vi "WPI_ADI_IMU_KalmanPitchRollYaw.vi"(6 "Reset?":bool, 7 "dt (ms)":dbl, 8 "Beta":dbl, 9 "Data":dbl[](array[numeric])) -> (3 "Output":dbl[](array[numeric]))   [LabVIEW 2015]
panel:
  out "output array":dbl[](array[numeric])
  out "Roll":dbl
  out "Pitch":dbl
  out "Yaw":dbl
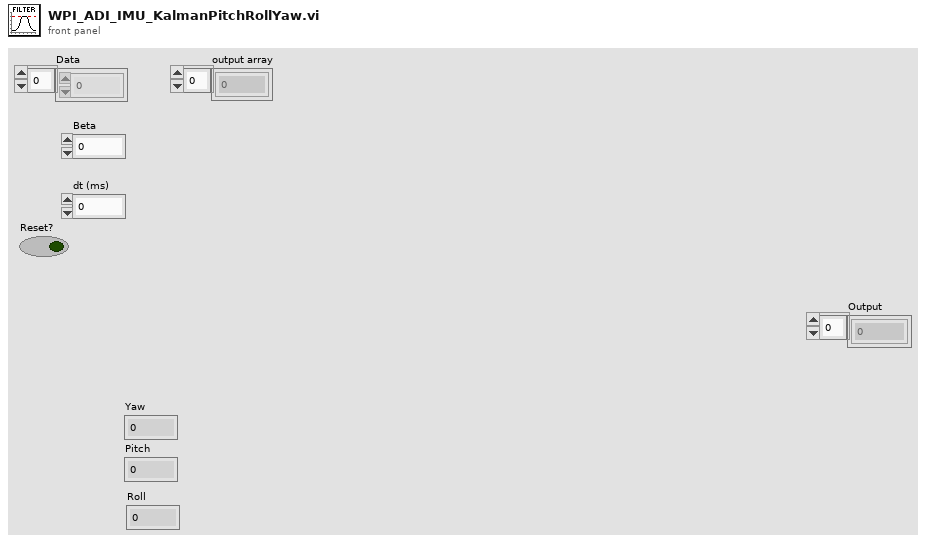
[diagram p1: front panel]
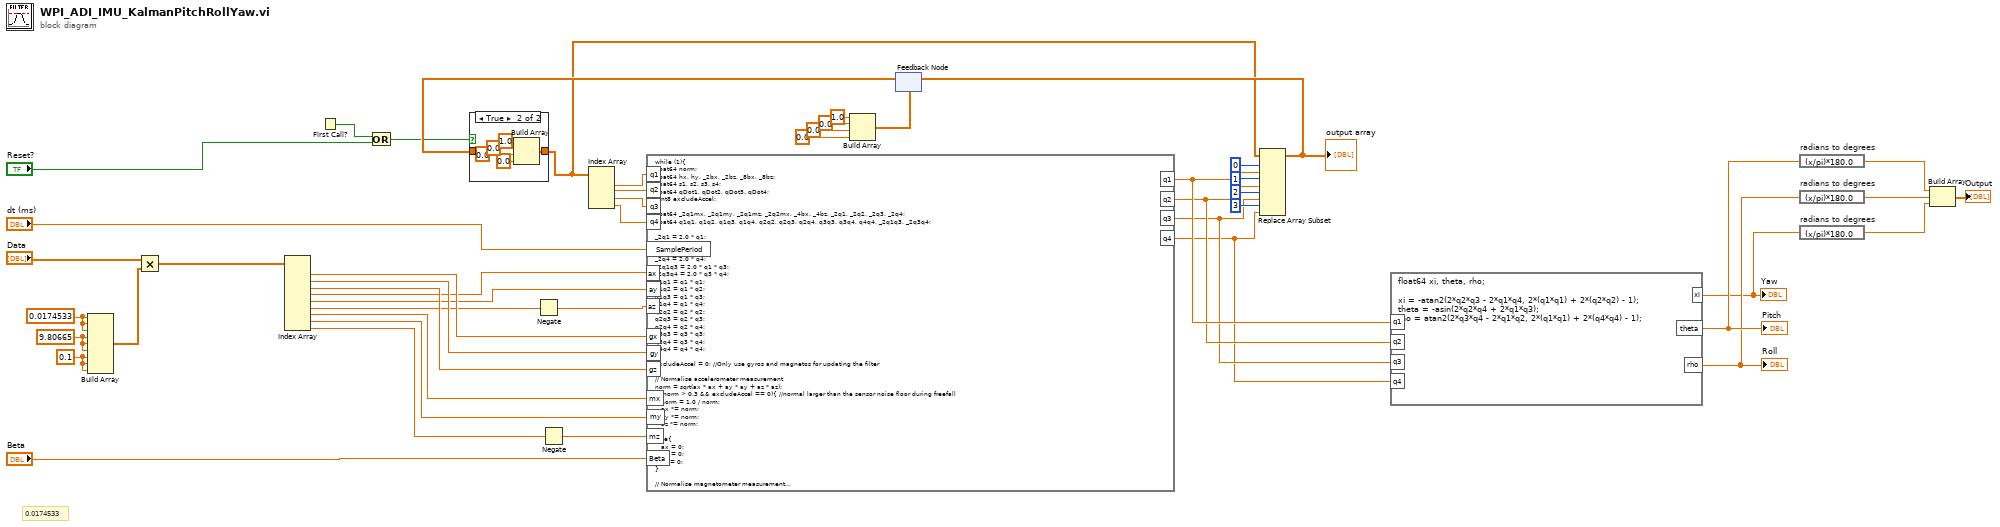
[diagram p0: block diagram]
diagram:
  w33 = 0.1
  w34 = 9.80665
  w35 = 0.0174533
  # "0.0174533"
  n1 = Build Array(w35, w35, w35, w34, w34, w34, w33, w33, w33) -> (w36:dbl[])
  n2 = Multiply(x="Data", y=w36) -> (x*y=w32:dbl[])
  n3 = Index Array(array=w32) -> (element #1=w49:dbl, element #2=w48:dbl, element #3=w47:dbl, element #4=w46:dbl, element #5=w45:dbl, element #6=w5:dbl, element #7=w1:dbl, element #8=w2:dbl, element #9=w4:dbl)  [unwired: 9 in]
  n4 = First Call?() -> (First Call?: T/F=w15:bool)
  n5 = Or(x=w15, y="Reset?") -> (x .or. y?=w16:bool)
  n6 = Negate(x=w5) -> (-x=w6:dbl)
  n7 = Negate(x=w4) -> (-x=w3:dbl)
  n8 = Build Array(1.0 ("element"), 0.0 ("element"), 0.0 ("element"), 0.0 ("element")) -> (w38:dbl[])
  n9 = feedback #1(w38) -> (w18:dbl[])
  n10 = case shown="True" w16 {
    tunnel: w18 -> [w50 _]
    tunnel: [w50 w51] -> w17
    frame False {
    }
    frame True {
      n11 = Build Array(1.0 ("element"), 0.0 ("element"), 0.0 ("element"), 0.0 ("element")) -> (w51:dbl[])
    }
  }
  n12 = Index Array(array=w17) -> (element #1=w31:dbl, element #2=w30:dbl, element #3=w29:dbl, element #4=w28:dbl)  [unwired: 4 in]
  n13 = formula code="while (1){\nfloat64 norm;\nfloat64 hx, hy, _2bx, _2bz, _8bx, _8bz;\nfloat64 s1, s2, s3, s4;\nfloat64 qDot1, qDot2, qDot3, qDot4;\nuInt8 excludeAccel;\n\nfloat64 _2q1mx, _2q1my, _2q1mz, _2q2mx, _4bx, _4bz, _2q1, _2q2, _2q3, _2q4;\nfloat64 q1q1, q1q2, q1q3, q1q4, q2q2, q2q3, q2q4, q3q3, q3q4, q4q4, _2q1q3, _2q3q4;\n\n_2q1 = 2.0 * q1;\n_2q2 = 2.0 * q2;\n_2q3 = 2.0 * q3;\n_2q4 = 2.0 * q4;\n_2q1q3 = 2.0 * q1 * q3;\n_2q3q4 = 2.0 * q3 * q4;\nq1q1 = q1 * q1;\nq1q2 = q1 * q2;\nq1q3 = q1 * q3;\nq1q4 = q1 * q4;\nq2q2 = q2 * q2;\nq2q3 = q2 * q3;\nq2q4 = q2 * q4;\nq3q3 = q3 * q3;\nq3q4 = q3 * q4;\nq4q4 = q4 * q4;\n\nexcludeAccel = 0; //Only use gyros and magnetos for updating the filter\n\n// Normalise accelerometer measurement\nnorm = sqrt(ax * ax + ay * ay + az * az);\nif (norm > 0.3 && excludeAccel == 0){ //normal larger than the sensor noise floor during freefall\n   norm = 1.0 / norm; \n   ax *= norm;\n   ay *= norm;\n   az *= norm;\n}\nelse{\n   ax = 0;\n   ay = 0;\n   az = 0;\n}\n\n// Normalise magnetometer measurement\nnorm = sqrt(mx * mx + my * my + mz * mz);\nif (norm > 0.0){\n   norm = 1.0 / norm;\n   mx *= norm;\n   my *= norm;\n   mz *= norm;\n}\nelse{\n  break; //something is wrong with the magneto readouts\n}\n\n// Reference direction of Earth's magnetic field\n_2q1mx = 2 * q1 * mx;\n_2q1my = 2 * q1 * my;\n_2q1mz = 2 * q1 * mz;\n_2q2mx = 2 * q2 * mx;\n\nhx = mx * q1q1 - _2q1my * q4 + _2q1mz * q3 + mx * q2q2 + _2q2 * my * q3 + _2q2 * mz * q4 - mx * q3q3 - mx * q4q4;\nhy = _2q1mx * q4 + my * q1q1 - _2q1mz * q2 + _2q2mx * q3 - my * q2q2 + my * q3q3 + _2q3 * mz * q4 - my * q4q4;\n_2bx = sqrt(hx * hx + hy * hy);\n_2bz = -_2q1mx * q3 + _2q1my * q2 + mz * q1q1 + _2q2mx * q4 - mz * q2q2 + _2q3 * my * q4 - mz * q3q3 + mz * q4q4;\n_4bx = 2.0 * _2bx;\n_4bz = 2.0 * _2bz;\n_8bx = 2.0 * _4bx;\n_8bz = 2.0 * _4bz;\n\n// Gradient descent algorithm corrective step\ns1 = -_2q3 * (2.0 * q2q4 - _2q1q3 - ax) + _2q2 * (2.0 * q1q2 + _2q3q4 - ay) - _4bz * q3 * (_4bx * (0.5 - q3q3 - q4q4) + _4bz * (q2q4 - q1q3) - mx) + (-_4bx * q4 + _4bz * q2) * (_4bx * (q2q3 - q1q4) + _4bz * (q1q2 + q3q4) - my) + _4bx * q3 * (_4bx * (q1q3 + q2q4) + _4bz * (0.5 - q2q2 - q3q3) - mz);\ns2 = _2q4 * (2.0 * q2q4 - _2q1q3 - ax) + _2q1 * (2.0 * q1q2 + _2q3q4 - ay) - 4.0 * q2 * (1.0 - 2.0 * q2q2 - 2.0 * q3q3 - az) + _4bz * q4 * (_4bx * (0.5 - q3q3 - q4q4) + _4bz * (q2q4 - q1q3) - mx) + (_4bx * q3 + _4bz * q1) * (_4bx * (q2q3 - q1q4) + _4bz * (q1q2 + q3q4) - my) + (_4bx * q4 - _8bz * q2) * (_4bx * (q1q3 + q2q4) + _4bz * (0.5 - q2q2 - q3q3) - mz);\ns3 = -_2q1 * (2.0 * q2q4 - _2q1q3 - ax) + _2q4 * (2.0 * q1q2 + _2q3q4 - ay) - 4.0 * q3 * (1.0 - 2.0 * q2q2 - 2.0 * q3q3 - az) + (-_8bx * q3 - _4bz * q1) * (_4bx * (0.5 - q3q3 - q4q4) + _4bz * (q2q4 - q1q3) - mx) + (_4bx * q2 + _4bz * q4) * (_4bx * (q2q3 - q1q4) + _4bz * (q1q2 + q3q4) - my) + (_4bx * q1 - _8bz * q3) * (_4bx * (q1q3 + q2q4) + _4bz * (0.5 - q2q2 - q3q3) - mz);\ns4 = _2q2 * (2.0 * q2q4 - _2q1q3 - ax) + _2q3 * (2.0 * q1q2 + _2q3q4 - ay) + (-_8bx * q4 + _4bz * q2) * (_4bx * (0.5 - q3q3 - q4q4) + _4bz * (q2q4 - q1q3) - mx) + (-_4bx * q1 + _4bz * q3) * (_4bx * (q2q3 - q1q4) + _4bz * (q1q2 + q3q4) - my) + _4bx * q2 * (_4bx * (q1q3 + q2q4) + _4bz * (0.5 - q2q2 - q3q3) - mz);\n\nnorm = sqrt(s1 * s1 + s2 * s2 + s3 * s3 + s4 * s4);\nif (norm > 0.0){\n   norm = 1.0 / norm;  //normalise gradient step\n   s1 *= norm;\n   s2 *= norm;\n   s3 *= norm;\n   s4 *= norm;\n}\nelse{\n   break;\n}\n\n// Compute rate of change of quaternion\nqDot1 = 0.5 * (-q2 * gx - q3 * gy - q4 * gz) - Beta * s1;\nqDot2 = 0.5 * (q1 * gx + q3 * gz - q4 * gy) - Beta * s2;\nqDot3 = 0.5 * (q1 * gy - q2 * gz + q4 * gx) - Beta * s3;\nqDot4 = 0.5 * (q1 * gz + q2 * gy - q3 * gx) - Beta * s4;\n\n// Integrate to yield quaternion\nq1 += qDot1 * SamplePeriod;\nq2 += qDot2 * SamplePeriod;\nq3 += qDot3 * SamplePeriod;\nq4 += qDot4 * SamplePeriod;\n\nnorm = sqrt(q1 * q1 + q2 * q2 + q3 * q3 + q4 * q4);\nif (norm > 0.0){\n   norm = 1.0 / norm;  //normalise quaternion\n   q1 = q1 * norm;\n   q2 = q2 * norm;\n   q3 = q3 * norm;\n   q4 = q4 * norm;\n}\nbreak;\n}"("q1"=w31, "gx"=w49, "gy"=w48, "gz"=w47, "ax"=w46, "ay"=w45, "az"=w6, "mx"=w1, "my"=w2, "mz"=w3, "SamplePeriod"="dt (ms)", "Beta"="Beta", "q2"=w30, "q3"=w29, "q4"=w28) -> ("q1"=w22:dbl, "q2"=w21:dbl, "q3"=w20:dbl, "q4"=w19:dbl)
  n14 = Replace Array Subset(array=w17, new element #1=w22, index #1=0 ("index"), new element #2=w21, index #2=1 ("index"), new element #3=w20, index #3=2 ("index"), new element #4=w19, index #4=3 ("index")) -> (w23:dbl[])
  "output array" <- w23
  n15 = feedback-in #1(w23) -> ()
  n16 = formula code="float64 xi, theta, rho;\n\nxi = -atan2(2*q2*q3 - 2*q1*q4, 2*(q1*q1) + 2*(q2*q2) - 1);\ntheta = -asin(2*q2*q4 + 2*q1*q3);\nrho = atan2(2*q3*q4 - 2*q1*q2, 2*(q1*q1) + 2*(q4*q4) - 1);"("q1"=w22, "q2"=w21, "q3"=w20, "q4"=w19) -> ("xi"=w11:dbl, "theta"=w13:dbl, "rho"=w12:dbl)
  "Yaw" <- w11
  "Pitch" <- w13
  "Roll" <- w12
  n17 = expression code="(x/pi)*180.0" "radians to degrees"(w13) -> (w10:dbl)
  n18 = expression code="(x/pi)*180.0" "radians to degrees"(w12) -> (w9:dbl)
  n19 = expression code="(x/pi)*180.0" "radians to degrees"(w11) -> (w8:dbl)
  n20 = Build Array(w10, w9, w8) -> (→"Output":dbl[])
